vi "Served_Global.vi"(0 "Mode":T1) -> (1 "Served VI Name":string[](array[string]), 2 "Served VI Path":path[](array[path]), 3 "Served IP Number & Port No":string[](array[string]))   [LabVIEW 2013]
uses:
  Controls/Serveds.ctl
  File/Setup_Filetype.ctl
  Preference_global.vi
  Constants_global.vi
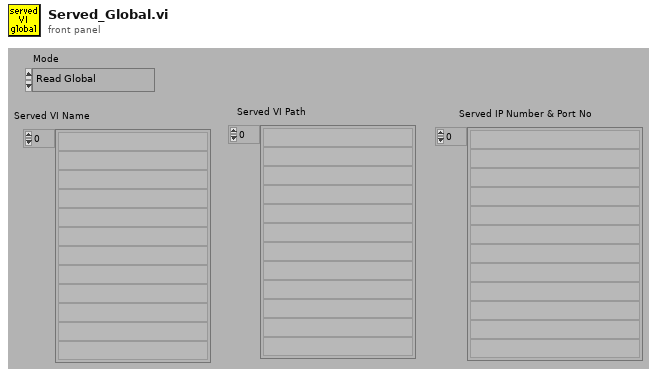
[diagram p1: front panel]
types:
  T1 = typedef "Serveds.ctl" = enum16{"Read Global", "Load Global From File"}
  T2 = typedef "Setup_Filetype.ctl" = enum16{"Measurement Setups", "Calibration Setups", "General", "Results File Plotter Setups", "Speed Calib Tweaks"}
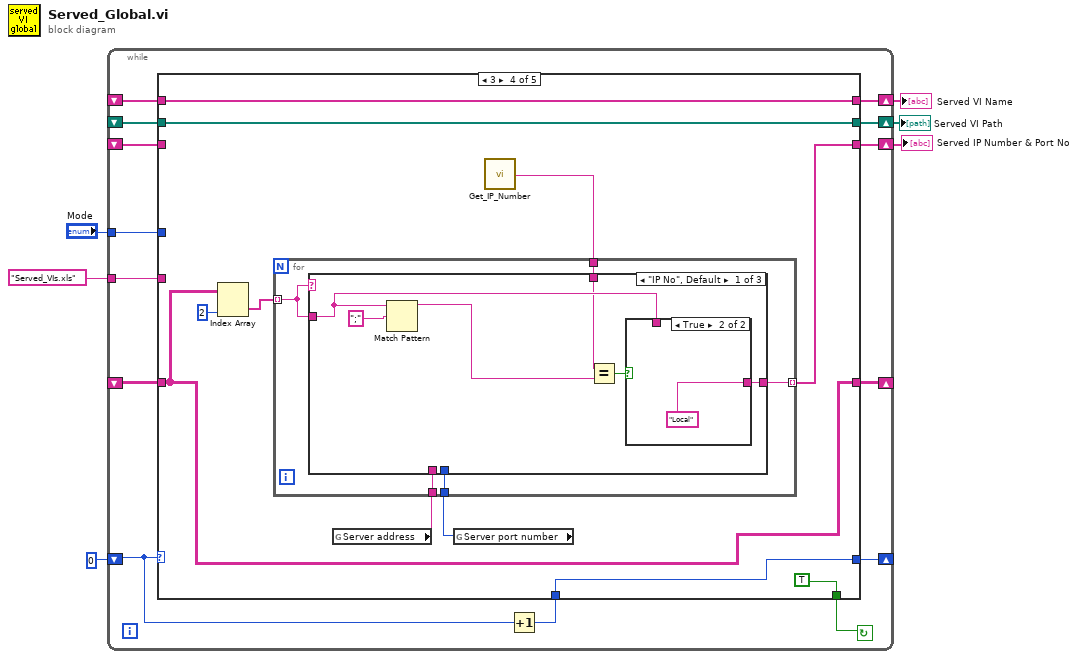
[diagram p0: block diagram]
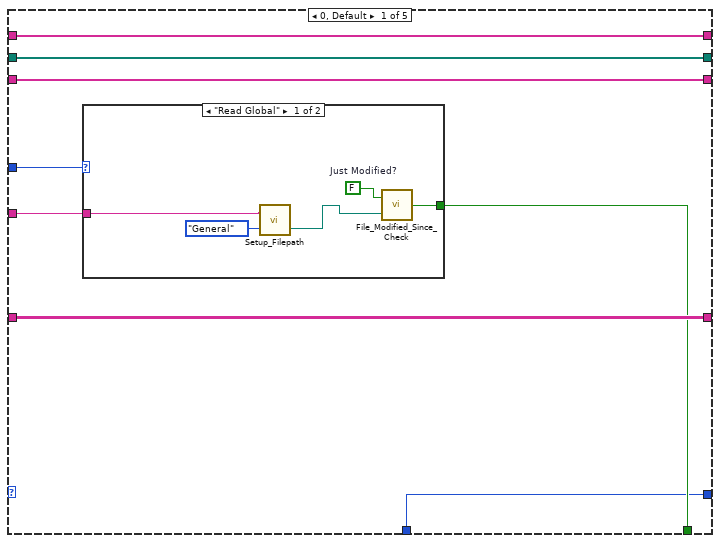
[diagram p2: hidden frame]
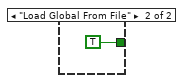
[diagram p3: hidden frame]
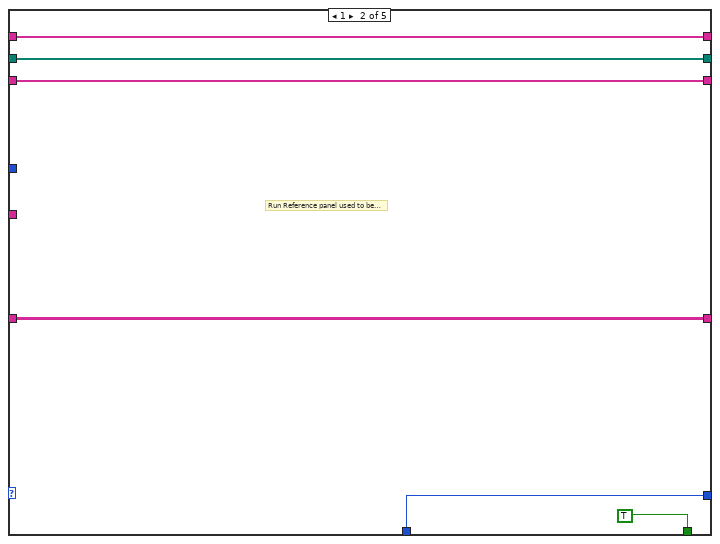
[diagram p4: hidden frame]
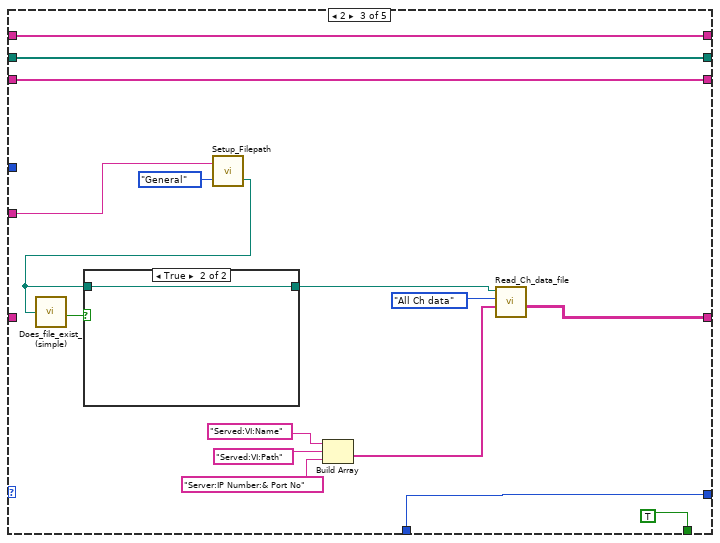
[diagram p5: hidden frame]
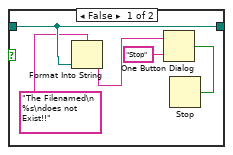
[diagram p6: hidden frame]
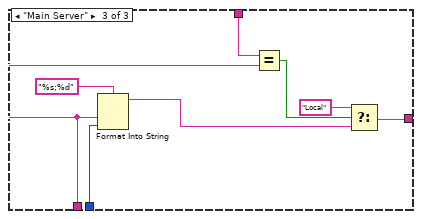
[diagram p9: hidden frame]
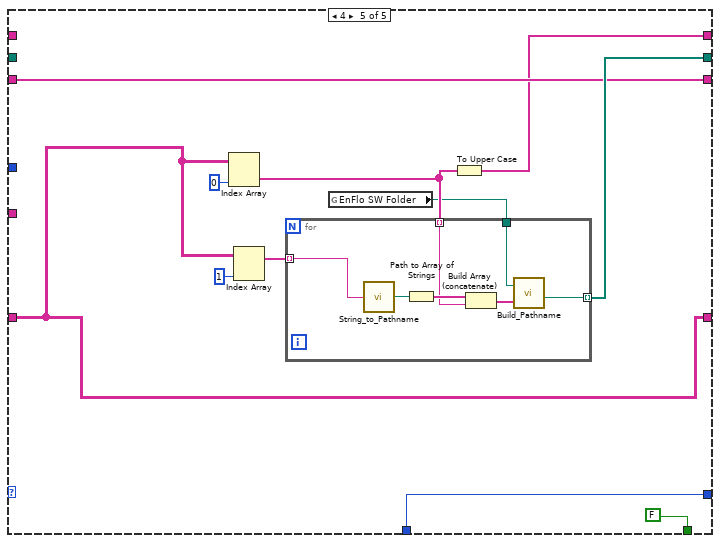
[diagram p10: hidden frame]
diagram:
  n1 = while {
    shift-left: _ -> [w8]
    shift-right: [w13] -> w4
    shift-left: _ -> [w12]
    shift-right: [w11] -> w3
    shift-left: _ -> [w10]
    shift-right: [w9] -> w2
    shift-left: _ -> [w16]
    shift-right: [w17] -> _
    tunnel: "Mode" -> [w18]
    shift-left: 0 -> [w15]
    shift-right: [w19] -> _
    tunnel: "Served_VIs.xls" ("Substring") -> [w7]
    stop <- w20 continue-if-true
    n2 = Increment(x=w15) -> (x+1=w14:i32)
    n3 = case shown="3" w15 {
      tunnel: [w26 TRUE TRUE TRUE FALSE] -> w20
      tunnel: [w25 w38 w51 w70 w105] -> w19
      tunnel: w18 -> [w27 _ _ _ _]
      tunnel: [w28 w40 w54 w67 w99] -> w17
      tunnel: w16 -> [w28 w40 _ w67 w99]
      tunnel: w14 -> [w25 w38 w51 w70 w105]
      tunnel: [w22 w35 w44 w68 w101] -> w13
      tunnel: w12 -> [w23 w36 w45 w65 _]
      tunnel: [w23 w36 w45 w65 w102] -> w11
      tunnel: w10 -> [w24 w37 w46 w64 _]
      tunnel: [w24 w37 w46 w64 w96] -> w9
      tunnel: w8 -> [w22 w35 w44 _ w101]
      tunnel: w7 -> [w21 _ w42 _ _]
      frame 0, Default {
        n4 = case shown="\"Read Global\"" w27 {
          tunnel: [w33 TRUE ("Modified?")] -> w26
          tunnel: w21 -> [w30 _]
          frame "Read Global" {
            w32 = FALSE  # Just Modified?
            n5 = call "Setup_Filepath.vi"("Setup File Type"=Setup_Filetype."General", "Filename in"=w30) -> ("Filename Out"=w29:path)  [unwired: 1 out]
            n6 = call "File_Modified_Since_Check.vi"("Pathname"=w29, "Just Modified?"=w32) -> ("Modified?"=w33:bool)
          }
          frame "Load Global From File" {
          }
        }
      }
      frame 1 {
        # "Run Reference panel used to be here"
      }
      frame 2 {
        n7 = call "Setup_Filepath.vi"("Setup File Type"=Setup_Filetype."General", "Filename in"=w42) -> ("Filename Out"=w41:path)  [unwired: 1 out]
        n8 = call "Does_file_exist_(simple).vi"("Pathname"=w41) -> ("exists?"=w53:bool)
        n9 = case shown="True" w53 {
          tunnel: w41 -> [w58 w62]
          tunnel: [w58 w62] -> w52
          frame False {
            n10 = Format Into String(format string="The Filenamed\n %s\ndoes not Exist!!" ("Format String"), w58) -> (resulting string=w60:string)  [unwired: 2 in, 1 out]
            n11 = One Button Dialog(message=w60, button name ("OK")="Stop") -> (true=w59:bool)
            n12 = Stop(stop? (T)=w59) -> ()
          }
          frame True {
          }
        }
        n13 = Build Array("Served:VI:Name", "Served:VI:Path", "Server:IP Number:& Port No") -> (w47:string[])
        n14 = call "Read_Ch_data_file.vi"("Present Channels"=w47, "Output"=enum16{"All Ch data", "The last few rows"}."All Ch data", "Filename"=w52) -> ("Channel Values"=w54:string[][])  [unwired: 2 in, 4 out]
      }
      frame 3 {
        n15 = Index Array(array=w67, index (col)=2) -> (element=w66:string[])  [unwired: 1 in]
        n16 = global read "Preference_global.vi" "Server address"() -> (w72:string)
        n17 = global read "Preference_global.vi" "Server port number"() -> (w71:u32)
        n18 = call "Get_IP_Number.vi"() -> ("IP Number"=w63:string)  [unwired: 1 out]
        n19 = for {
          tunnel: [w78] -> w68 mode=indexing
          tunnel: w72 -> [w77]
          tunnel: w71 -> [w76]
          tunnel: w63 -> [w75]
          tunnel: w66 -> [w74] mode=indexing
          n20 = case shown="\"IP No\", Default" w74 {
            tunnel: [w83 w87 w88] -> w78
            tunnel: w77 -> [_ _ w92]
            tunnel: w76 -> [_ _ w95]
            tunnel: w74 -> [w81 w87 _]
            tunnel: w75 -> [w79 _ w93]
            frame "IP No", Default {
              n21 = Match Pattern(string=w81, regular expression=";") -> (before substring=w80:string)  [unwired: 4 out]
              n22 = Equal?(x=w79, y=w80) -> (x = y?=w82:bool)
              n23 = case shown="True" w82 {
                tunnel: [w85 "Local" ("t")] -> w83
                tunnel: w81 -> [w85 _]
                frame False {
                }
                frame True {
                }
              }
            }
            frame "Local" {
            }
            frame "Main Server" {
              n24 = Format Into String(format string="%s;%d" ("Format String"), w92, w95) -> (resulting string=w90:string)  [unwired: 2 in, 1 out]
              n25 = Equal?(x=w93, y=w92) -> (x = y?=w91:bool)
              n26 = Select(t="Local", s=w91, f=w90) -> (s? t:f=w88:string)
            }
          }
        }
      }
      frame 4 {
        n27 = Index Array(array=w99, index (col)=0 ("Index")) -> (element=w98:string[])  [unwired: 1 in]
        n28 = Index Array(array=w99, index (col)=1 ("Index")) -> (element=w103:string[])  [unwired: 1 in]
        n29 = global read "Constants_global.vi" "EnFlo SW Folder"() -> (w97:path)
        n30 = for {
          tunnel: w103 -> [w113] mode=indexing
          tunnel: [w107] -> w102 mode=indexing
          tunnel: w98 -> [w110] mode=indexing
          tunnel: w97 -> [w109]
          n31 = call "String_to_Pathname.vi"("Input String"=w113) -> ("path"=w112:path)
          n32 = Path to Array of Strings(0:w112) -> (2:w111:string[])  [unwired: 1 out]
          n33 = Build Array (concatenate)(w111, w110) -> (w108:string[])
          n34 = call "Build_Pathname.vi"("PathElements"=w108, "PathnameIn"=w109) -> ("AppendedPath"=w107:path)
        }
        n35 = To Upper Case(1:w98) -> (0:w96:string[])
      }
    }
  }
  "Served IP Number & Port No" <- w4
  "Served VI Name" <- w2
  "Served VI Path" <- w3
